vi "Set Ctl Params.vi"(8 "error in (no error)":errorcluster, 10 "Ctl Params":cluster{"htx":dbl, "clx":dbl}, 11 "TE Cooler in":refnum<class "TE Cooler.lvclass">) -> (0 "error out":errorcluster, 3 "TE Cooler out":refnum<class "TE Cooler.lvclass">)   [LabVIEW 2015, in "TE Cooler.lvlib" / "TE Cooler.lvclass"]
doc: "Update two of the more important control parameters in both the object and on the controller: the heat side multiplier (htx) and the cool side multiplier (clx). These two values control how much power is applied when the TE Cooler is cooling or heating (values range from 0 to 2)."
uses:
  TE Cooler.lvclass
  Controls/Command.ctl
  TE Cooler.lvclass/TE Cooler.ctl
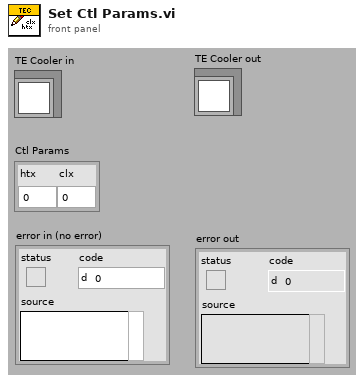
[diagram p1: front panel]
types:
  T1 = typedef "TE Cooler.lvlib/TE Cooler.lvclass/Command.ctl" = enum16{"INPUT1", "DESIRED CONTROL VALUE", "POWER OUTPUT", "ALARM STATUS", "INPUT 2", "OUTPUT CURRENT COUNTS", "ALARM TYPE", "SET TYPE DEFINE", "SENSOR TYPE", "CONTROL TYPE", "CONTROL OUTPUT POLARITY", "POWER ON/OFF", "OUTPUT SHUTDOWN IF ALARM", "FIXED DESIRED CONTROL SETTING", "PROPORTIONAL BANDWIDTH", "INTEGRAL GAIN", "DERIVATIVE GAIN", "LOW EXTERNAL SET RANGE", "HIGH EXTERNAL SET RANGE", "ALARM DEADBAND", "HIGH ALARM SETTING", "LOW ALARM SETTING", "CONTROL DEADBAND SETTING", "INPUT1 OFFSET", "INPUT2 OFFSET", "HEAT MULTIPLIER", "COOL MULTIPLIER", "OVER CURRENT COUNT COMPARE VALUE", "ALARM LATCH ENABLE", "NOT USED", "ALARM LATCH RESET", "CHOOSE SENSOR FOR ALARM FUNCTION", "CHOOSE TEMPERATURE WORKING UNITS", "EEPROM WRITE ENABLE", "OVER CURRENT CONTINUOUS", "OVER CURRENT RESTART ATTEMPTS", "JP3 DISPLAY ENABLE"}
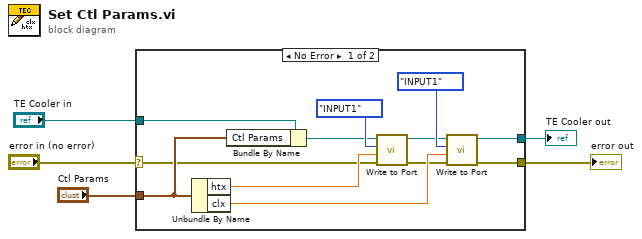
[diagram p0: block diagram]
diagram:
  n1 = case shown="No Error" "error in (no error)" {
    selector: "error in (no error)" -> [w8 w18]
    tunnel: [w6 w18] -> w4
    tunnel: [w13 w19] -> w2
    tunnel: "TE Cooler in" -> [w14 w19]
    tunnel: "Ctl Params" -> [w11 _]
    frame No Error {
      n2 = Unbundle By Name(w11) -> ("htx"=w10:dbl, "clx"=w9:dbl)
      n3 = Bundle By Name(cluster=w14, "Ctl Params"=w11) -> (w12:refnum<class "TE Cooler.lvclass">)
      n4 = call "Write to Port.vi"("error in"=w8, "Input Value"=w10, "TEC Cmd"=Command."INPUT1", "TE Cooler in"=w12) -> ("error out"=w7:errorcluster, "TE Cooler out"=w15:refnum<class "TE Cooler.lvclass">)  [unwired: 5 in, 1 out]
      n5 = call "Write to Port.vi"("error in"=w7, "Input Value"=w9, "TEC Cmd"=Command."INPUT1", "TE Cooler in"=w15) -> ("error out"=w6:errorcluster, "TE Cooler out"=w13:refnum<class "TE Cooler.lvclass">)  [unwired: 5 in, 1 out]
    }
    frame Error {
    }
  }
  "error out" <- w4
  "TE Cooler out" <- w2
